vi "MPM_Get_Enable_Module.vi"(8 "error in (no error)":errorcluster, 11 ".NET Reference in":refnum<k24>) -> (0 "error out":errorcluster, 2 "enableModules":i32[](array[numeric]), 3 "Reference out":refnum<k24>)   [LabVIEW 2017]
uses:
  D:/test/FULLband-sts/Fullband_Sample/DLL/InstrumentDLL.dll
  DLL/InstrumentDLL.dll
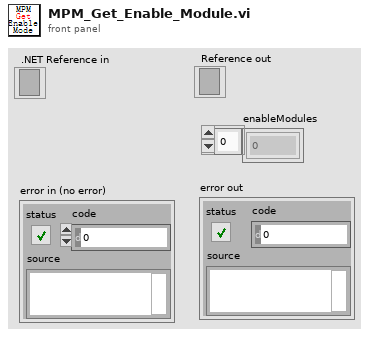
[diagram p1: front panel]
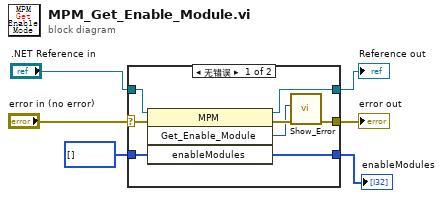
[diagram p0: block diagram]
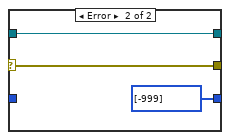
[diagram p2: hidden frame]
diagram:
  n1 = case shown="无错误" "error in (no error)" {
    selector: "error in (no error)" -> [w12 w16]
    tunnel: ".NET Reference in" -> [w14 w17]
    tunnel: [w13 w17] -> w5
    tunnel: [w11 w16] -> w3
    tunnel: [w8 i32[] [-999] ("enableModules")] -> w2
    tunnel: i32[] [] ("enableModules") -> [w7 _]
    frame No Error {
      n2 = invoke class="MPM" method="Get_Enable_Module"(reference=w14, error in=w12, "enableModules"=w7) -> (reference out=w13:refnum<k24>, error out=w10:errorcluster, "Get_Enable_Module"=w9:i32, "enableModules"=w8:i32[])  [unwired: 1 in]
      n3 = call "Show_Error.vi"("error in (no error)"=w10, "Error"=w9) -> ("error out"=w11:errorcluster)  [unwired: 9 in]
    }
    frame Error {
    }
  }
  "Reference out" <- w5
  "error out" <- w3
  "enableModules" <- w2
